vi "Drive Controller.vi"(8 "error in":errorcluster) -> ()   [LabVIEW 2019]
doc: "This VI executes continuously carrying out the current operation and responding to updates or new operation requests. It will often contain the timing or control code that is difficult to place directly in TeleOp. This VI generally opens all sensors and motors and isolates the rest of the robot code from knowing implementation details of how the operations are carried out."
uses:
  <vilib>/Rock Robotics/WPI/Framework/Completion Status.ctl
  Drive Setpoints.ctl
  Drive Operations.ctl
  <vilib>/Rock Robotics/WPI/ThirdParty/Phoenix-LabVIEW/Motor Controller/Controls/CTRE_Phoenix_MotorControl_ControlMode.ctl
  <vilib>/Rock Robotics/WPI/Gyro/WPI_GyroDevRef.ctl
  <vilib>/Rock Robotics/SystemInterfaces/AI/FPGA_AIChannel.ctl
  <vilib>/Rock Robotics/SystemInterfaces/spilib/spi_bus.ctl
  CAN Functions/TalonSRX6Motor.ctl
  <vilib>/Rock Robotics/WPI/MotorControl/WPI_MotorControlDeviceRef.ctl
  <vilib>/Rock Robotics/WPI/MotorControl/WPI_MotorControlType.ctl
  <vilib>/Rock Robotics/SystemInterfaces/DIO/FPGA_DIOPWMChannel.ctl
  <vilib>/Rock Robotics/WPI/PWM/WPI_PWMDeadband.ctl
  <vilib>/Rock Robotics/SystemInterfaces/DIO/FPGA_DIOChannel.ctl
  <vilib>/Platform/TimedLoop/XDataNode/timing_clust.ctl
  <vilib>/Platform/TimedLoop/XDataNode/nitl_modes.ctl
  <vilib>/Platform/TimedLoop/XDataNode/wakeup.ctl
  Odometry/Typedef/Odometry.ctl
  Pure Pursuit/Typedef/Pure Pursuit Telemetry.ctl
  Pure Pursuit/Typedef/Path Point.ctl
  Is High Gear.vi
  <vilib>/platform/TimedLoop/XDataNode/XDataNode.xnode
  <vilib>/Platform/TimedLoop/XDataNode/XDNodeRunTimeDep.lvlib
  <vilib>/ptbypt/NI_PtbyPt.lvlib
  Pure Pursuit/Pure Pursuit.lvlib
  <vilib>/Analysis/NI_AALPro.lvlib
panel:
  in  "Tab Control":T1(tab)
  in  "Interactive Values":T2
  out "Setpoints":T4(graph)
  in  "Buttons":cluster{"Execute Cmd":bool, "Abort Cmd":bool}
  out "Command Timing":cluster{"Start Time (ms)":u32, "Iterations":i32}
  out "Status":T5
  in  "PIDF gains":cluster{"Kp":dbl, "Ki":dbl, "Kd":dbl, "Kf":dbl}={"Kp"=7.5, "Ki"=0.05, "Kd"=2.5, "Kf"=0.0} caption="PIDF gains (turn to angle only)" {"Kf" format="%.3f"; "Kd" format="%.5f"; "Ki" format="%.5f"; "Kp" format="%.5f"}
  in  "Control Mode":T6 caption="Control Mode (Teleop only)" items=["PercentOutput"=0, "Position"=1, "Velocity"=2, "Current"=3, "Follower"=5, "MotionProfile"=6, "MotionMagic"=7, "MotionProfileArc"=10, "Disabled"=15]
  in  "i Zone":dbl=8.0 format="%.2f"
  in  "Trackwidth":dbl=25.0 format="%#_13g"
  in  "Max Velocity":dbl=400.0
  in  "Max Accel":dbl=2500.0
  in  "Lookahead":dbl=18.0
  in  "kffv":dbl
  in  "kffa":dbl=3.0
  in  "Velocity Offset High Gear":dbl
  in  "Velocity Offset Low Gear":dbl=0.08
  in  "Value":dbl
  in  "Run":bool
  out "Waveform Chart":dbl(graph)
  out "XY Graph":cluster{"X":dbl, "Y":dbl}[](graph)
  in  "Test":string(combo)="quasi-static ramp"
  out "Path":cluster{dbl[], dbl[]}[](graph)
  in  "Points to Follow":cluster{dbl[], dbl[]}={[0.0, 40.0, 60.0, 100.0], [0.0, 20.0, 80.0, 40.0]}
  in  "Type of Interpolation":T7(ring)=enum."Spline"
  in  "Interpolation factor (n)":i32(slide)=100 scale=0.0..20.0
  in  "Build and set Path":bool
  out "Current\nCmd":string
  # "Interactive Command: You may fill in the settings for a command\nand schedule it with the Execute button. You can observe and abort\nany command while fine tuning the code for the controller."
  # "Pure Pursuit"
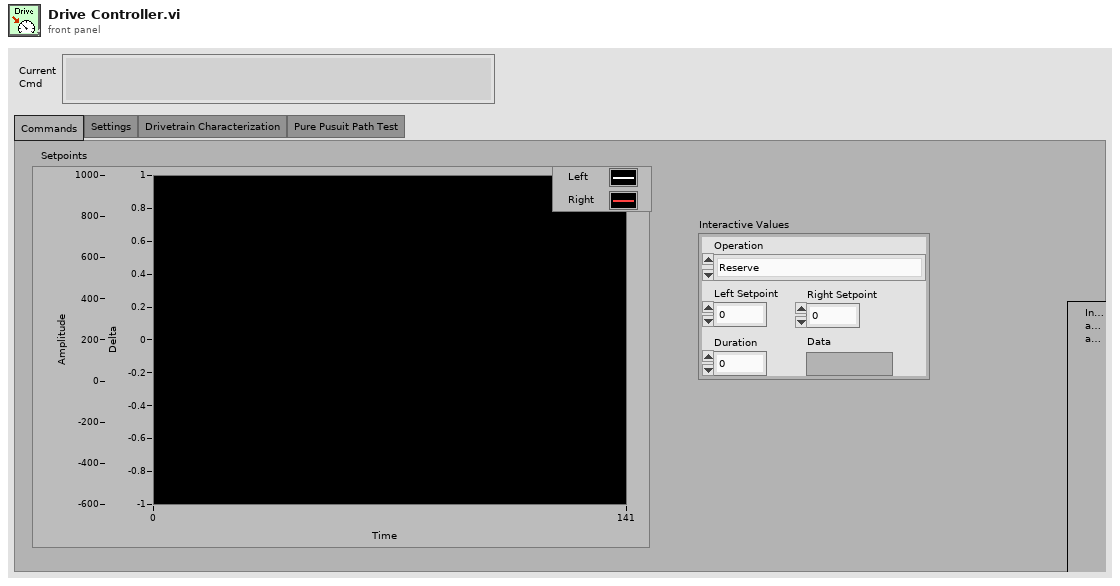
[diagram p1: front panel]
types:
  T1 = enum32{"Commands", "Settings", "Drivetrain Characterization", "Pure Pusuit Path Test"}
  T2 = typedef "Drive Setpoints.ctl" = cluster{"Operation":T3, "Left Setpoint":dbl, "Right Setpoint":dbl, "Duration":dbl, "Data":variant}
  T3 = typedef "Drive Operations.ctl" = enum16{"Reserve", "Read Current", "Immediate", "Drive for Time", "Drive for Distance", "Turn to Angle", "Drivetrain Char", "Pure Pursuit"}
  T4 = cluster{"Don't move motors while reserved":dbl, "Don't move motors while reserved":dbl, "Left Velocity Raw":i32, "Right Velocity Raw":i32, i32}
  T5 = typedef "Completion Status.ctl" = enum16{"Successful", "Aborted", "Incomplete"}
  T6 = typedef "CTRE_Phoenix_MotorControl_ControlMode.ctl" = u16
  T7 = enum16{"Linear", "Polynomial", "Spline", "Rational"}
  T8 = typedef "WPI_GyroDevRef.ctl" = cluster{"DevStatus":errorcluster, "Analog Channel":T9, "Gain (VoltsPerDegree/Second)":dbl, "Gyro Type":enum16{"Analog", "XRS450"}, "Handle":i32, "SPI Bus":T10, "Device Found":bool, "Sample Rate":dbl, "Calibrate On Open":bool, "Offset":dbl}
  T9 = typedef "FPGA_AIChannel.ctl" = enum8{"AI 0", "AI 1", "AI 2", "AI 3", "AI MXP 0", "AI MXP 1", "AI MXP 2", "AI MXP 3", "Invalid"}
  T10 = typedef "spi_bus.ctl" = enum16{"SPI On-Board, CS0", "SPI On-Board, CS1", "SPI On-Board, CS2", "SPI On-Board, CS3", "SPI MXP", "Invalid"}
  T11 = typedef "TalonSRX6Motor.ctl" = cluster{"FrontLeftMaster":T12, "FrontLeftSlave1":T12, "FrontLeftSlave2":T12, "FrontRightMaster":T12, "FrontRightSlave1":T12, "FrontRightSlave2":T12}
  T12 = typedef "WPI_MotorControlDeviceRef.ctl" = cluster{"DeviceStatus":errorcluster, "Type":T13, "PWM":cluster{"PWM Channel":T14, "DeadBand":T15}, "CAN":cluster{"Device Number":u8, "SetOutput VI Ref":variant, "GetOutput VI Ref":variant, "Enable VI Ref":variant, "Disable VI Ref":variant, "Data":variant}, "Invert":bool, "DIO PWM":cluster{"PWM \"Enable\" Channel":T14, "DIOChannel":T16, "PWM Rate":dbl}}
  T13 = typedef "WPI_MotorControlType.ctl" = enum16{"PWM", "CAN", "DIO PWM"}
  T14 = typedef "FPGA_DIOPWMChannel.ctl" = enum8{"PWM 0", "PWM 1", "PWM 2", "PWM 3", "PWM 4", "PWM 5", "PWM 6", "PWM 7", "PWM 8", "PWM 9", "PWM MXP 0", "PWM MXP 1", "PWM MXP 2", "PWM MXP 3", "PWM MXP 4", "PWM MXP 5", "PWM MXP 6", "PWM MXP 7", "PWM MXP 8", "PWM MXP 9", "Invalid"}
  T15 = typedef "WPI_PWMDeadband.ctl" = cluster{"Name":string, "maxPositivePwm":i32, "minPositivePwm":i32, "centerPwm":i32, "maxNegativePwm":i32, "minNegativePwm":i32, "angularRange":u16}
  T16 = typedef "FPGA_DIOChannel.ctl" = enum8{"DIO 0", "DIO 1", "DIO 2", "DIO 3", "DIO 4", "DIO 5", "DIO 6", "DIO 7", "DIO 8", "DIO 9", "DIO MXP 0", "DIO MXP 1", "DIO MXP 2", "DIO MXP 3", "DIO MXP 4", "DIO MXP 5", "DIO MXP 6", "DIO MXP 7", "DIO MXP 8", "DIO MXP 9", "DIO MXP 10", "DIO MXP 11", "DIO MXP 12", "DIO MXP 13", "DIO MXP 14", "DIO MXP 15", "SPI Port CS1", "SPI Port CS2", "SPI Port CS3", "SPI Port MISO", "SPI Port MOSI", "Invalid"}
  T17 = typedef "XDNodeRunTimeDep.lvlib/timing_clust.ctl" = cluster{"Expected End [f-1]":u64, "Actual End [f-1]":u64, "Finished Late? [f-1]":bool, "Expected End [i-1]":u64, "Actual End [i-1]":u64, "Finished Late? [i-1]":bool, "Expected Start [i]":u64, "Actual Start [i]":u64, "Expected Start [f]":u64, "Actual Start [f]":u64, "Source Name":string, "Structure Name":string, "Period":i64, "Deadline":i64, "Offset":i64, "Start":i64, "Priority":i32, "Timeout":i32, "Mode":T18, "Wakeup Reason":T19, "Error":errorcluster, "Source Type":string, "Secondary Source Type":string, "Global End Time":u64, "Global Start Time":u64, "Frame Duration":u64, "Iteration Duration":u64, "Assigned CPU":i32, "I/O Scan Engine Mode":u32}
  T18 = typedef "XDNodeRunTimeDep.lvlib/nitl_modes.ctl" = enum32{"No Change", "Process missed periods, maintain original phase", "Discard missed periods, maintain original phase", "Process missed periods, ignore original phase", "Discard missed periods, ignore original phase"}
  T19 = typedef "XDNodeRunTimeDep.lvlib/wakeup.ctl" = enum32{"Normal", "Aborted", "Asynchronous wakeup", "Timing source error", "Timed loop error", "Timeout"}
  T20 = typedef "Command Status Info.ctl" = cluster{"Name":string, "Status":T5, "notifier out":T21}
  T21 = typedef "Completion Notifier.ctl" = refnum<notifier>
  T22 = cluster{"SubSystem Data":T2, cluster{"Start Time (ms)":u32, "Iterations":i32}, cluster{"Command Info":T20, "Description":string, "Default Command":T2, "queue out":refnum<queue>, "Subsystem Name":string}}
  T23 = typedef "Pure Pursuit.lvlib/Pure Pursuit Telemetry.ctl" = cluster{"Target Point":T24, "Close Point":T24, "Curvature":dbl, "index out":i32}
  T24 = typedef "Pure Pursuit.lvlib/Path Point.ctl" = cluster{"x":dbl, "y":dbl, "heading":dbl, "curvature":dbl, "total distance":dbl, "velocity expected":dbl}
  T25 = typedef "Odometry.ctl" = cluster{"x":dbl, "y":dbl, "theta":dbl, "Left Encoder Raw":i32, "Right Encoder Raw":i32, "Left Velocity Raw":i32, "Right Velocity Raw":i32, "Left Encoder":dbl, "Right Encoder":dbl, "Late Iterations":i16}
  T26 = cluster{"SubSystem Data":T2, cluster{"Start Time (ms)":u32, "Iterations":i32}, "Default Command Arguments":cluster{"Command Info":T20, "Description":string, "Default Command":T2, "queue out":refnum<queue>, "Subsystem Name":string}}
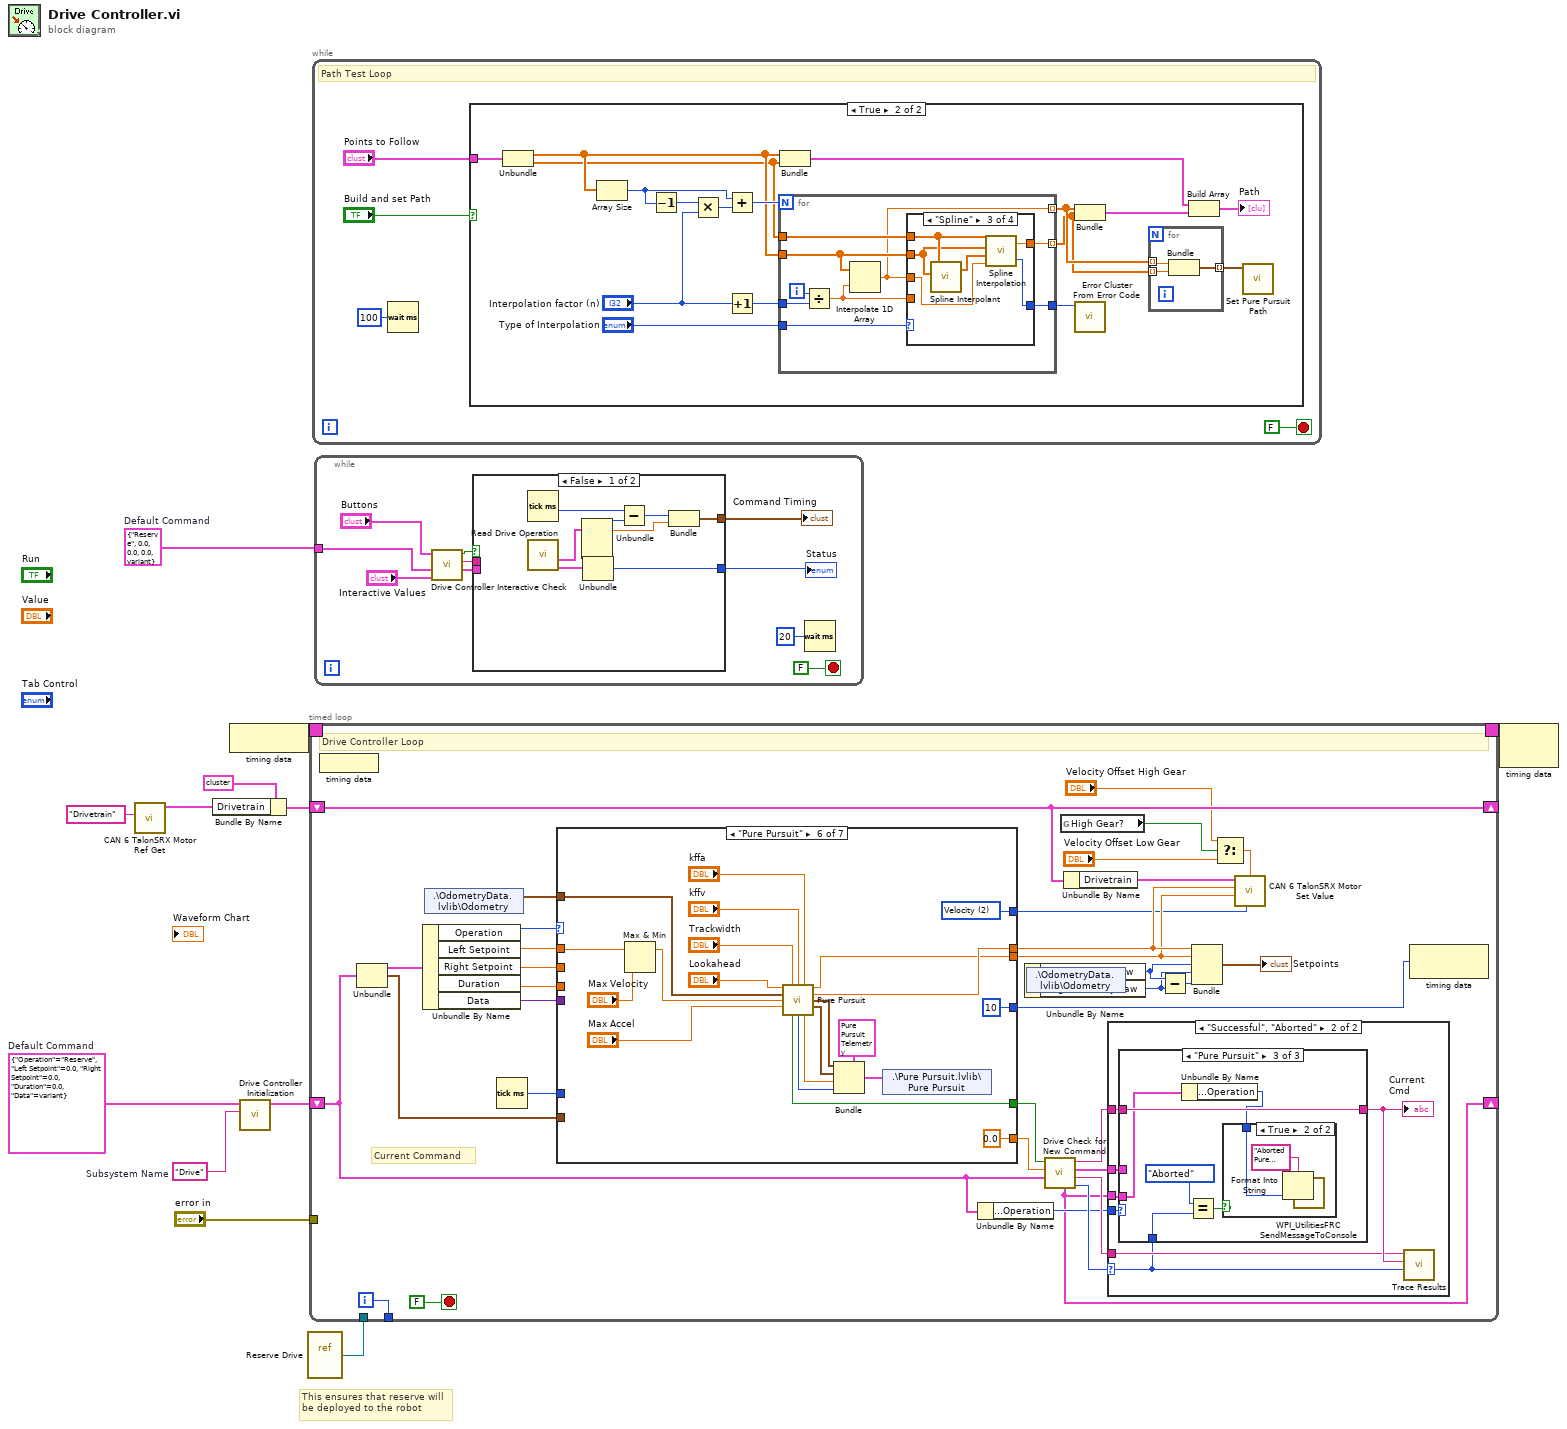
[diagram p0: block diagram]
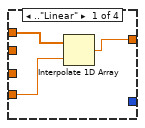
[diagram p3: hidden frame]
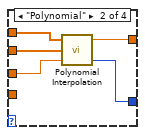
[diagram p4: hidden frame]
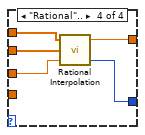
[diagram p5: hidden frame]
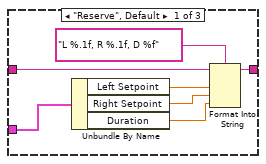
[diagram p7: hidden frame]
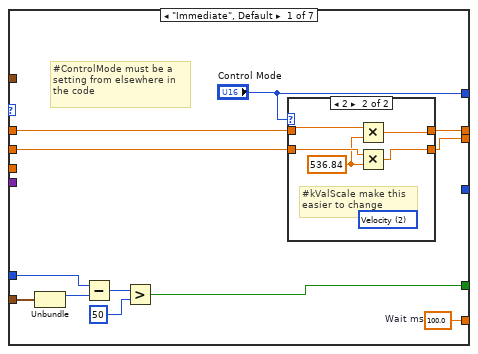
[diagram p10: hidden frame]
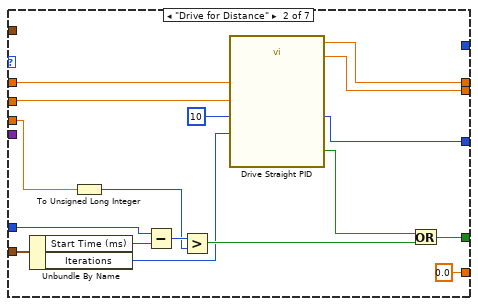
[diagram p12: hidden frame]
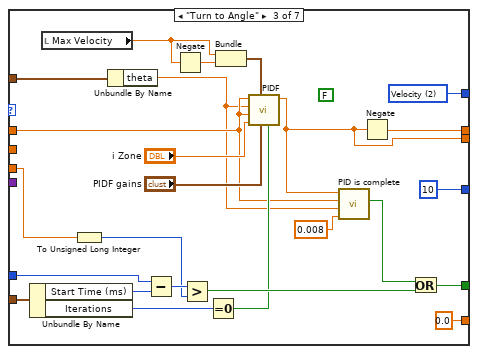
[diagram p13: hidden frame]
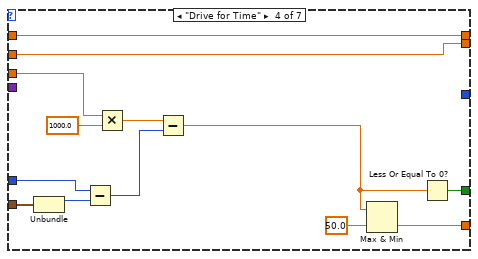
[diagram p14: hidden frame]
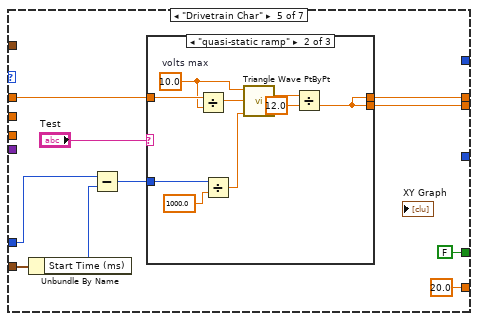
[diagram p15: hidden frame]
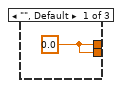
[diagram p16: hidden frame]
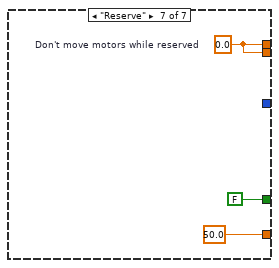
[diagram p18: hidden frame]
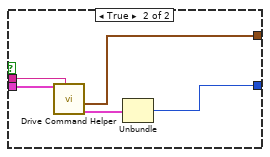
[diagram p19: hidden frame]
diagram:
  w5 = T2 {"Operation"=enum."Reserve", "Left Setpoint"=0.0, "Right Setpoint"=0.0, "Duration"=0.0, "Data"=variant}  # Default Command
  w8 = T2 {"Operation"=enum."Reserve", "Left Setpoint"=0.0, "Right Setpoint"=0.0, "Duration"=0.0, "Data"=variant}  # Default Command
  w12 = "Drive"  # Subsystem Name
  # "This ensures that reserve will\nbe deployed to the robot"
  n1 = call "CAN 6 TalonSRX Motor Ref Get.vi"("refnum name"="Drivetrain") -> ("TalonSRX6MotorRef out"=w1:T11)  [unwired: 9 in, 1 out]
  n2 = Bundle By Name(cluster=cluster{"Gyro":T8, "Drivetrain":T11} {"Gyro"={"DevStatus"={"status"=FALSE, "code"=0, "source"=""}, "Analog Channel"=enum."Invalid", "Gain (VoltsPerDegree/Second)"=0.0, "Gyro Type"=enum."Analog", "Handle"=0, "SPI Bus"=enum."Invalid", "Device Found"=FALSE, "Sample Rate"=1.0, "Calibrate On Open"=FALSE, "Offset"=0.0}, "Drivetrain"={"FrontLeftMaster"={"DeviceStatus"={"status"=FALSE, "code"=0, "source"=""}, "Type"=enum."PWM", "PWM"={"PWM Channel"=enum."PWM 1", "DeadBand"={"Name"="", "maxPositivePwm"=0, "minPositivePwm"=0, "centerPwm"=0, "maxNegativePwm"=0, "minNegativePwm"=0, "angularRange"=0}}, "CAN"={"Device Number"=0, "SetOutput VI Ref"=variant(enum8{"Percent VBus", "Current", "Speed", "Position", "Voltage"} enum."Percent VBus"), "GetOutput VI Ref"=variant(refnum<k1> refnum), "Enable VI Ref"=variant(dbl 12.0), "Disable VI Ref"=variant(enum8{"Percent VBus", "Speed", "Position", "Slave", "Unchanged / Invalid", "Voltage Compensation", "Current", "Motion Profile"} enum."Percent VBus"), "Data"=variant}, "Invert"=FALSE, "DIO PWM"={"PWM \"Enable\" Channel"=enum."Invalid", "DIOChannel"=enum."Invalid", "PWM Rate"=0.0}}, "FrontLeftSlave1"={"DeviceStatus"={"status"=FALSE, "code"=0, "source"=""}, "Type"=enum."PWM", "PWM"={"PWM Channel"=enum."PWM 1", "DeadBand"={"Name"="", "maxPositivePwm"=0, "minPositivePwm"=0, "centerPwm"=0, "maxNegativePwm"=0, "minNegativePwm"=0, "angularRange"=0}}, "CAN"={"Device Number"=0, "SetOutput VI Ref"=variant(enum8{"Percent VBus", "Current", "Speed", "Position", "Voltage"} enum."Percent VBus"), "GetOutput VI Ref"=variant(refnum<k1> refnum), "Enable VI Ref"=variant(dbl 12.0), "Disable VI Ref"=variant(enum8{"Percent VBus", "Speed", "Position", "Slave", "Unchanged / Invalid", "Voltage Compensation", "Current", "Motion Profile"} enum."Percent VBus"), "Data"=variant}, "Invert"=FALSE, "DIO PWM"={"PWM \"Enable\" Channel"=enum."Invalid", "DIOChannel"=enum."Invalid", "PWM Rate"=0.0}}, "FrontLeftSlave2"={"DeviceStatus"={"status"=FALSE, "code"=0, "source"=""}, "Type"=enum."PWM", "PWM"={"PWM Channel"=enum."PWM 1", "DeadBand"={"Name"="", "maxPositivePwm"=0, "minPositivePwm"=0, "centerPwm"=0, "maxNegativePwm"=0, "minNegativePwm"=0, "angularRange"=0}}, "CAN"={"Device Number"=0, "SetOutput VI Ref"=variant(enum8{"Percent VBus", "Current", "Speed", "Position", "Voltage"} enum."Percent VBus"), "GetOutput VI Ref"=variant(refnum<k1> refnum), "Enable VI Ref"=variant(dbl 12.0), "Disable VI Ref"=variant(enum8{"Percent VBus", "Speed", "Position", "Slave", "Unchanged / Invalid", "Voltage Compensation", "Current", "Motion Profile"} enum."Percent VBus"), "Data"=variant}, "Invert"=FALSE, "DIO PWM"={"PWM \"Enable\" Channel"=enum."Invalid", "DIOChannel"=enum."Invalid", "PWM Rate"=0.0}}, "FrontRightMaster"={"DeviceStatus"={"status"=FALSE, "code"=0, "source"=""}, "Type"=enum."PWM", "PWM"={"PWM Channel"=enum."PWM 1", "DeadBand"={"Name"="", "maxPositivePwm"=0, "minPositivePwm"=0, "centerPwm"=0, "maxNegativePwm"=0, "minNegativePwm"=0, "angularRange"=0}}, "CAN"={"Device Number"=0, "SetOutput VI Ref"=variant(enum8{"Percent VBus", "Current", "Speed", "Position", "Voltage"} enum."Percent VBus"), "GetOutput VI Ref"=variant(refnum<k1> refnum), "Enable VI Ref"=variant(dbl 12.0), "Disable VI Ref"=variant(enum8{"Percent VBus", "Speed", "Position", "Slave", "Unchanged / Invalid", "Voltage Compensation", "Current", "Motion Profile"} enum."Percent VBus"), "Data"=variant}, "Invert"=FALSE, "DIO PWM"={"PWM \"Enable\" Channel"=enum."Invalid", "DIOChannel"=enum."Invalid", "PWM Rate"=0.0}}, "FrontRightSlave1"={"DeviceStatus"={"status"=FALSE, "code"=0, "source"=""}, "Type"=enum."PWM", "PWM"={"PWM Channel"=enum."PWM 1", "DeadBand"={"Name"="", "maxPositivePwm"=0, "minPositivePwm"=0, "centerPwm"=0, "maxNegativePwm"=0, "minNegativePwm"=0, "angularRange"=0}}, "CAN"={"Device Number"=0, "SetOutput VI Ref"=variant(enum8{"Percent VBus", "Current", "Speed", "Position", "Voltage"} enum."Percent VBus"), "GetOutput VI Ref"=variant(refnum<k1> refnum), "Enable VI Ref"=variant(dbl 12.0), "Disable VI Ref"=variant(enum8{"Percent VBus", "Speed", "Position", "Slave", "Unchanged / Invalid", "Voltage Compensation", "Current", "Motion Profile"} enum."Percent VBus"), "Data"=variant}, "Invert"=FALSE, "DIO PWM"={"PWM \"Enable\" Channel"=enum."Invalid", "DIOChannel"=enum."Invalid", "PWM Rate"=0.0}}, "FrontRightSlave2"={"DeviceStatus"={"status"=FALSE, "code"=0, "source"=""}, "Type"=enum."PWM", "PWM"={"PWM Channel"=enum."PWM 1", "DeadBand"={"Name"="", "maxPositivePwm"=0, "minPositivePwm"=0, "centerPwm"=0, "maxNegativePwm"=0, "minNegativePwm"=0, "angularRange"=0}}, "CAN"={"Device Number"=0, "SetOutput VI Ref"=variant(enum8{"Percent VBus", "Current", "Speed", "Position", "Voltage"} enum."Percent VBus"), "GetOutput VI Ref"=variant(refnum<k1> refnum), "Enable VI Ref"=variant(dbl 12.0), "Disable VI Ref"=variant(enum8{"Percent VBus", "Speed", "Position", "Slave", "Unchanged / Invalid", "Voltage Compensation", "Current", "Motion Profile"} enum."Percent VBus"), "Data"=variant}, "Invert"=FALSE, "DIO PWM"={"PWM \"Enable\" Channel"=enum."Invalid", "DIOChannel"=enum."Invalid", "PWM Rate"=0.0}}}}, "Drivetrain"=w1) -> (w3:cluster{"Gyro":T8, "Drivetrain":T11})
  n3 = node-c288() -> (w7:T17)
  n4 = call "Drive Controller Initialization.vi"("Subsystem Name"=w12, "Default Command"=w8) -> ("Current Command"=w10:T22)  [unwired: 9 in]
  n5 = vi-ref "Reserve Drive.vi"() -> (w9:refnum<vi>)
  n6 = timed-loop {
    shift-right: [w22] -> _
    shift-left: w10 -> [w31]
    tunnel: [w46] -> _
    tunnel: "error in" -> [_]
    tunnel: w9 -> [_]
    timing: w7 -> [_]
    timing-out: [_] -> w6
    shift-right: [w29] -> _
    shift-left: w3 -> [w29]
    i -> [w46]
    stop <- FALSE stop-if-true
    # "Current Command"
    # "Drive Controller Loop"
    n7 = node-c288() -> ()  [unwired: 1 in]
    n8 = Unbundle(w31) -> ("SubSystem Data"=w45:T2, w34:cluster{"Start Time (ms)":u32, "Iterations":i32})  [unwired: 1 out]
    n9 = Unbundle By Name(w45) -> ("Operation"=w44:T3, "Left Setpoint"=w43:dbl, "Right Setpoint"=w42:dbl, "Duration"=w41:dbl, "Data"=w23:variant)
    n10 = shared-variable ".\\OdometryData.lvlib\\Odometry"() -> (w24:T25)  [unwired: 1 in, 1 out]
    n11 = Tick Count (ms)() -> (millisecond timer value=w40:u32)
    n12 = case shown="\"Pure Pursuit\"" w44 {
      tunnel: [w87 0.0 ("Wait ms") 0.0 ("Wait ms") w137 20.0 ("Wait ms") 0.0 ("Wait ms") 50.0] -> w33
      tunnel: [w82 w102 w130 w143 FALSE ("ignore previous (F)") w188 FALSE ("ignore previous (F)")] -> w38
      tunnel: w34 -> [w81 w109 w134 w145 w154 _ _]
      tunnel: [w77 w106 w112 w142 w157 w177 w191] -> w28
      tunnel: [w76 w105 w111 w141 w156 w176 w191] -> w27
      tunnel: w43 -> [w79 w101 w120 w142 w155 w175 _]
      tunnel: w42 -> [w78 w100 _ w141 _ _ _]
      tunnel: w41 -> [_ w97 w128 w136 _ _ _]
      tunnel: w40 -> [w83 w108 w133 w140 w152 _ _]
      tunnel: [_ w98 i64 10 ("Period") _ _ i64 10 ("Period") _] -> w32
      tunnel: ["Control Mode" _ w116 _ _ w190 _] -> w16
      tunnel: w24 -> [_ _ w118 _ _ w185 _]
      tunnel: w23 -> [_ _ _ _ _ _ _]
      frame "Immediate", Default {
        w87 = 100.0  # Wait ms
        # "#ControlMode must be a\nsetting from elsewhere in \nthe code"
        n13 = Unbundle(w81) -> ("Start Time (ms)"=w84:u32)  [unwired: 1 out]
        n14 = Subtract(x=w83, y=w84) -> (x-y=w85:u32)
        n15 = Greater?(x=w85, y=u32 50 ("Left Motor")) -> (0:w82:bool)
        n16 = case shown="2" "Control Mode" {
          tunnel: w79 -> [w89 w94]
          tunnel: w78 -> [w88 w92]
          tunnel: [w89 w93] -> w77
          tunnel: [w88 w91] -> w76
          frame 0, Default {
          }
          frame 2 {
            w90 = 536.84 ("y")
            (unwired) T6 2 items=["PercentOutput"=0, "Position"=1, "Velocity"=2, "Current"=3, "Follower"=5, "MotionProfile"=6, "MotionMagic"=7, "MotionMagicArc"=8, "MotionProfileArc"=10, "Disabled"=15] ("Control Mode")
            # "#kValScale make this\neasier to change"
            n17 = Multiply(x=w94, y=w90) -> (x*y=w93:dbl)
            n18 = Multiply(x=w92, y=w90) -> (x*y=w91:dbl)
          }
        }
      }
      frame "Drive for Distance" {
        w98 = i64 10 ("Period")
        n19 = Unbundle By Name(w109) -> ("Start Time (ms)"=w96:u32, "Iterations"=w99:i32)
        n20 = To Unsigned Long Integer(number=w97) -> (unsigned 32bit integer=w95:u32)
        n21 = Subtract(x=w108, y=w96) -> (x-y=w107:u32)
        n22 = Greater?(x=w107, y=w95) -> (0:w103:bool)
        n23 = call "Drive Straight PID.vi"("Angle Offset"=w100, "Iteration"=w99, "target distance"=w101, "Period (ms)"=w98) -> ("Complete?"=w104:bool, "Right Axis"=w105:dbl, "Left Axis"=w106:dbl)  [unwired: 5 in]
        n24 = Or(x=w104, y=w103) -> (x .or. y?=w102:bool)
      }
      frame "Turn to Angle" {
        w116 = T6 2 items=["PercentOutput"=0, "Position"=1, "Velocity"=2, "Current"=3, "Follower"=5, "MotionProfile"=6, "MotionMagic"=7, "MotionMagicArc"=8, "MotionProfileArc"=10, "Disabled"=15] ("Control Mode")
        (unwired) FALSE ("Square Inputs")
        n25 = Unbundle By Name(w134) -> ("Start Time (ms)"=w127:u32, "Iterations"=w123:i32)
        n26 = local read "Max Velocity"() -> (w114:dbl)
        n27 = To Unsigned Long Integer(number=w128) -> (unsigned 32bit integer=w126:u32)
        n28 = Unbundle By Name(w118) -> ("theta"=w117:dbl)
        n29 = Subtract(x=w133, y=w127) -> (x-y=w132:u32)
        n30 = Negate(x=w114) -> (-x=w113:dbl)
        n31 = Greater?(x=w132, y=w126) -> (0:w131:bool)
        n32 = Equal To 0?(x=w123) -> (x = 0?=w122:bool)
        n33 = Bundle("Max Velocity"=w114, w113) -> (w115:cluster{"Max Velocity":dbl, dbl})  [unwired: 1 in]
        n34 = call "PIDF.vi"("reinitialize? (F)"=w122, "PIDF gains"="PIDF gains", "output range"=w115, "i Zone"="i Zone", "Feedforward"=w120, "process variable"=w117, "setpoint"=w120) -> ("output"=w111:dbl)  [unwired: 2 in, 2 out]
        n35 = call "PID is complete.vi"("threshold"=0.008, "process variable"=w117, "setpoint"=w120, "PID Output"=w111) -> ("PID is Done?"=w121:bool)  [unwired: 6 in, 1 out]
        n36 = Negate(x=w111) -> (-x=w112:dbl)
        n37 = Or(x=w121, y=w131) -> (x .or. y?=w130:bool)
      }
      frame "Drive for Time" {
        n38 = Unbundle(w145) -> ("Start Time (ms)"=w144:u32)  [unwired: 1 out]
        n39 = Subtract(x=w140, y=w144) -> (x-y=w148:u32)
        n40 = Multiply(x=w136, y=1000.0) -> (x*y=w147:dbl)
        n41 = Subtract(x=w147, y=w148) -> (x-y=w139:dbl)
        n42 = Max & Min(x=w139, y=50.0) -> (min(x,y)=w137:dbl)  [unwired: 1 out]
        n43 = Less Or Equal To 0?(x=w139) -> (x <= 0?=w143:bool)
      }
      frame "Drivetrain Char" {
        n44 = Unbundle By Name(w154) -> ("Start Time (ms)"=w153:u32)
        n45 = Subtract(x=w152, y=w153) -> (x-y=w151:u32)
        n46 = case shown="\"quasi-static ramp\"" "Test" {
          tunnel: [w159 w162 w169] -> w157
          tunnel: [w159 w162 w169] -> w156
          tunnel: w155 -> [_ w164 w169]
          tunnel: w151 -> [_ w168 _]
          frame "", Default {
            w159 = 0.0
          }
          frame "quasi-static ramp" {
            w161 = 10.0  # volts max
            n47 = Divide(x=w164, y=w161) -> (x/y=w165:dbl)
            n48 = Divide(x=w168, y=1000.0 ("amplitude")) -> (x/y=w167:dbl)
            n49 = call <vilib>:"Triangle Wave PtByPt.vi"("time"=w167, "frequency"=w165, "amplitude"=w161) -> ("triangle wave"=w163:dbl)  [unwired: 1 in]
            n50 = Divide(x=w163, y=12.0) -> (x/y=w162:dbl)
          }
          frame "step-voltage acceleration" {
          }
        }
      }
      frame "Pure Pursuit" {
        w190 = T6 2 items=["PercentOutput"=0, "Position"=1, "Velocity"=2, "Current"=3, "Follower"=5, "MotionProfile"=6, "MotionMagic"=7, "MotionMagicArc"=8, "MotionProfileArc"=10, "Disabled"=15] ("Control Mode")
        n51 = Max & Min(x=w175, y="Max Velocity") -> (max(x,y)=w173:dbl)  [unwired: 1 out]
        n52 = call "Pure Pursuit.vi"("Lookahead"="Lookahead", "Trackwidth"="Trackwidth", "kffv"="kffv", "kffa"="kffa", "Odometry"=w185, "Max Velocity"=w173, "Max Accel"="Max Accel") -> ("Left Velocity"=w176:dbl, "Right Velocity"=w177:dbl, "Target Point"=w182:T24, "Close Point"=w181:T24, "Finished?"=w188:bool, "index out"=w170:i32, "Curvature"=w180:dbl)  [unwired: 1 in, 1 out]
        n53 = Bundle(cluster=T23 {"Target Point"={"x"=0.0, "y"=0.0, "heading"=0.0, "curvature"=0.0, "total distance"=0.0, "velocity expected"=0.0}, "Close Point"={"x"=0.0, "y"=0.0, "heading"=0.0, "curvature"=0.0, "total distance"=0.0, "velocity expected"=0.0}, "Curvature"=0.0, "index out"=0} ("Pure Pursuit"), "Target Point"=w182, "Close Point"=w181, "Curvature"=w180, "index out"=w170) -> (w171:T23)
        n54 = shared-variable ".\\Pure Pursuit.lvlib\\Pure Pursuit"(w171) -> ()  [unwired: 1 in, 1 out]
      }
      frame "Reserve" {
        w191 = 0.0  # Don't move motors while reserved
      }
    }
    n55 = Unbundle By Name(w31) -> ("SubSystem Data.Operation"=w30:T3)
    n56 = shared-variable ".\\OdometryData.lvlib\\Odometry"() -> (w17:T25)  [unwired: 1 in, 1 out]
    n57 = Unbundle By Name(w17) -> ("Left Velocity Raw"=w15:i32, "Right Velocity Raw"=w14:i32)
    n58 = call "Drive Check for New Command.vi"("input cluster"=w31, "Wait time (ms)"=w33, "Finished?"=w38) -> ("Completion"=w39:T5, "Subsystem Name"=w35:string, "Current Command"=w36:T2, "Initial Trace String"=w37:string, "Next Command"=w22:T26)  [unwired: 4 in]
    n59 = global read "Is High Gear.vi" "High Gear?"() -> (w20:bool)
    n60 = Unbundle By Name(w29) -> ("Drivetrain"=w25:T11)
    n61 = case shown="\"Successful\", \"Aborted\"" w39 {
      selector: w39 -> [_ w53]
      tunnel: w37 -> [_ w57]
      tunnel: w36 -> [_ w58]
      tunnel: w35 -> [_ w55]
      tunnel: w30 -> [_ w54]
      tunnel: w22 -> [_ w52]
      frame "Incomplete", Default {
        # "Continuing current command"
      }
      frame "Successful", "Aborted" {
        # "Report and setup for next command"
        n62 = case shown="\"Pure Pursuit\"" w54 {
          tunnel: w58 -> [w62 _ _]
          tunnel: w57 -> [w61 w66 w72]
          tunnel: [w60 w66 w72] -> w56
          tunnel: w53 -> [_ _ w71]
          tunnel: w52 -> [_ _ w68]
          frame "Reserve", Default {
            n63 = Unbundle By Name(w62) -> ("Left Setpoint"=w64:dbl, "Right Setpoint"=w65:dbl, "Duration"=w59:dbl)
            n64 = Format Into String(format string="L %.1f, R %.1f, D %f", initial string=w61, w64, w65, w59) -> (resulting string=w60:string)  [unwired: 1 in, 1 out]
          }
          frame "Read Current" {
            # "Placeholder for \ncomplex commands\nwith cleanup"
          }
          frame "Pure Pursuit" {
            n65 = Unbundle By Name(w68) -> ("SubSystem Data.Operation"=w67:T3)
            n66 = Equal?(x=Completion_Status."Aborted", y=w71) -> (x = y?=w69:bool)
            n67 = case shown="True" w69 {
              tunnel: w67 -> [_ w73]
              frame False {
              }
              frame True {
                n68 = Format Into String(format string="Aborted Pure Pursuit for: %s", w73) -> (resulting string=w75:string)  [unwired: 2 in, 1 out]
                n69 = call <vilib>:"WPI_UtilitiesFRC SendMessageToConsole.vi"("Message"=w75) -> ()  [unwired: 14 in, 1 out]
              }
            }
          }
        }
        "Current\nCmd" <- w56
        n70 = call <vilib>:"Trace Results.vi"("Status of previous command"=w53, "Description"=w56, "Subsystem"=w55) -> ()  [unwired: 9 in]
      }
    }
    n71 = Subtract(x=w15, y=w14) -> (x-y=w13:i32)
    n72 = Bundle("Don't move motors while reserved"=w28, "Don't move motors while reserved"=w27, "Left Velocity Raw"=w15, "Right Velocity Raw"=w14, w13) -> (→"Setpoints":T4)  [unwired: 1 in]
    n73 = Select(t="Velocity Offset High Gear", s=w20, f="Velocity Offset Low Gear") -> (s? t:f=w18:dbl)
    n74 = call "CAN 6 TalonSRX Motor Set Value.vi"("Control Mode"=w16, "Velocity Offset"=w18, "Right Power"=w27, "Left Power"=w28, "Drivetrain"=w25) -> ()  [unwired: 7 in]
    n75 = node-c288(w32) -> ()  [unwired: 1 out]
  }
  n76 = while {
    stop <- FALSE stop-if-true
    # "Path Test Loop"
    n77 = Wait (ms)(milliseconds to wait=u32 100) -> ()  [unwired: 1 out]
    n78 = case shown="True" "Build and set Path" {
      tunnel: "Points to Follow" -> [_ w206]
      frame False {
      }
      frame True {
        n79 = Unbundle(w206) -> (w205:dbl[], w204:dbl[])
        n80 = Array Size(array=w205) -> (size(s)=w209:i32)
        n81 = Decrement(x=w209) -> (x-1=w212:i32)
        n82 = Multiply(x=w212, y="Interpolation factor (n)") -> (x*y=w210:i32)
        n83 = Add(x=w209, y=w210) -> (x+y=w208:i32)
        n84 = Increment(x="Interpolation factor (n)") -> (x+1=w211:i32)
        n85 = for {
          N: w208 -> [_]
          tunnel: w204 -> [w226]
          tunnel: w205 -> [w220]
          tunnel: [w225] -> w207
          tunnel: "Type of Interpolation" -> [w221]
          tunnel: w211 -> [w223]
          tunnel: [w222] -> w202 mode=indexing
          tunnel: [w219] -> w203 mode=indexing
          i -> [w224]
          n86 = Divide(x=w224, y=w223) -> (x/y=w218:dbl)
          n87 = Interpolate 1D Array(1:w218, 2:w220) -> (0:w219:dbl)
          n88 = case shown="\"Spline\"" w221 {
            tunnel: w219 -> [_ w234 w237 w241]
            tunnel: [w228 w233 w235 w243] -> w222
            tunnel: [_ w232 w236 w242] -> w225
            tunnel: w220 -> [_ w231 w238 w244]
            tunnel: w226 -> [w229 w230 w240 w245]
            tunnel: w218 -> [w227 _ _ _]
            frame .."Linear" {
              n89 = Interpolate 1D Array(1:w227, 2:w229) -> (0:w228:dbl)
            }
            frame "Polynomial" {
              n90 = call <vilib>:"Polynomial Interpolation.vi"("x value"=w234, "X"=w231, "Y"=w230) -> ("error"=w232:i32, "interpolation value"=w233:dbl)  [unwired: 1 out]
            }
            frame "Spline" {
              n91 = call <vilib>:"Spline Interpolant.vi"("X"=w238, "Y"=w240) -> ("Interpolant"=w239:dbl[])  [unwired: 2 in, 1 out]
              n92 = call <vilib>:"Spline Interpolation.vi"("x value"=w237, "Interpolant"=w239, "X"=w238, "Y"=w240) -> ("error"=w236:i32, "interpolation value"=w235:dbl)
            }
            frame "Rational".. {
              n93 = call <vilib>:"Rational Interpolation.vi"("x value"=w241, "X"=w244, "Y"=w245) -> ("error"=w242:i32, "interpolation value"=w243:dbl)  [unwired: 1 out]
            }
          }
        }
        n94 = Bundle(w205, w204) -> (w201:cluster{dbl[], dbl[]})  [unwired: 1 in]
        n95 = Bundle(w203, w202) -> (w200:cluster{dbl[], dbl[]})  [unwired: 1 in]
        n96 = call <vilib>:"Error Cluster From Error Code.vi"("error code (0)"=w207) -> ()  [unwired: 8 in, 1 out]
        n97 = for {
          tunnel: w203 -> [w217] mode=indexing
          tunnel: w202 -> [w216] mode=indexing
          tunnel: [w215] -> w198 mode=indexing
          n98 = Bundle(w217, "interpolation value"=w216) -> (w215:cluster{dbl, "interpolation value":dbl})  [unwired: 1 in]
        }
        n99 = Build Array(w201, w200) -> (→"Path":cluster{dbl[], dbl[]}[])
        n100 = call "Set Pure Pursuit Path.vi"("Path"=w198) -> ()  [unwired: 10 in, 1 out]
      }
    }
  }
  n101 = while {
    tunnel: w5 -> [w247]
    stop <- FALSE stop-if-true
    n102 = call "Drive Controller Interactive Check.vi"("Interactive Command In"="Interactive Values", "Default Command"=w247, "Buttons"="Buttons") -> ("Interactive Command Out"=w249:T2, "Trace String"=w250:string, "Schedule"=w251:bool)  [unwired: 6 in]
    n103 = case shown="False" w251 {
      tunnel: [w260 w268] -> w252
      tunnel: [w259 w264] -> w253
      tunnel: w250 -> [_ w266]
      tunnel: w249 -> [_ w265]
      frame False {
        n104 = Tick Count (ms)() -> (millisecond timer value=w263:u32)
        n105 = call "Read Drive Operation.vi"() -> ("Command Info"=w257:T20, "SubSystem Data"=w256:T2)  [unwired: 9 in, 1 out]
        n106 = Unbundle(w256) -> ("Operation"=w261:T3, "Left Setpoint"=w258:dbl)  [unwired: 3 out]
        n107 = Unbundle(w257) -> ("Status"=w260:T5)  [unwired: 2 out]
        n108 = Subtract(x=w263, y=w261) -> (x-y=w262:u32)
        n109 = Bundle(w262, "Left Setpoint"=w258) -> (w259:cluster{u32, "Left Setpoint":dbl})  [unwired: 1 in]
      }
      frame True {
        n110 = call "Drive Command Helper.vi"("Description"=w266, "SubSystem Data"=w265) -> ("Command Info Out"=w267:T20, "Command Timing"=w264:cluster{"Start Time (ms)":u32, "Iterations":i32})  [unwired: 7 in, 1 out]
        n111 = Unbundle(w267) -> ("Status"=w268:T5)  [unwired: 2 out]
      }
    }
    "Status" <- w252
    "Command Timing" <- w253
    n112 = Wait (ms)(milliseconds to wait=u32 20) -> ()  [unwired: 1 out]
  }
  n113 = node-c288(w6) -> ()  [unwired: 1 out]
